vi "Read Test.vi"() -> ()   [LabVIEW 2020]
uses:
  <vilib>/Waveform/WDTOps.llb/WDT Get Waveform Time Array DBL.vi
panel:
  out "x-y 2":dbl
  out "x-y":dbl
  out "XY Graph":cluster{"X array":timestamp[], "Y":dbl[]}(graph)
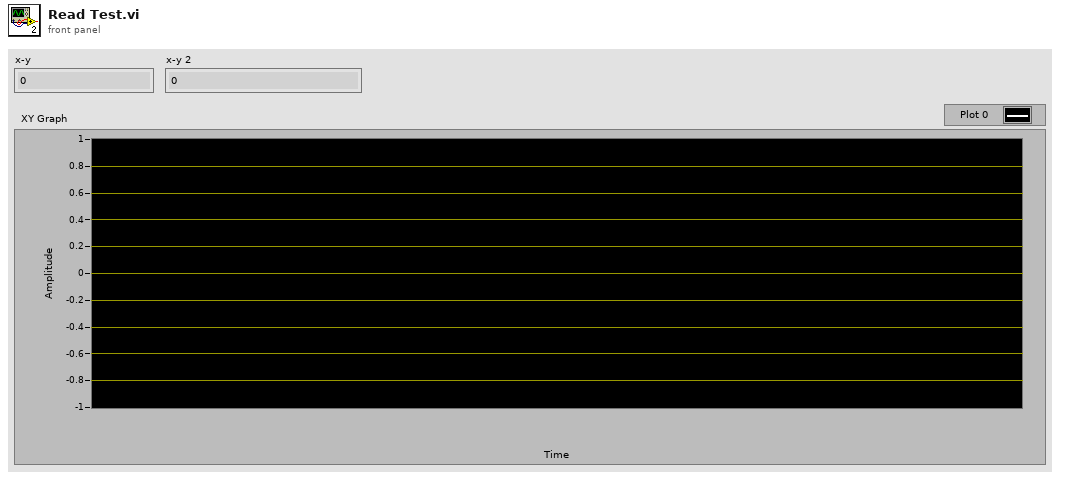
[diagram p1: front panel]
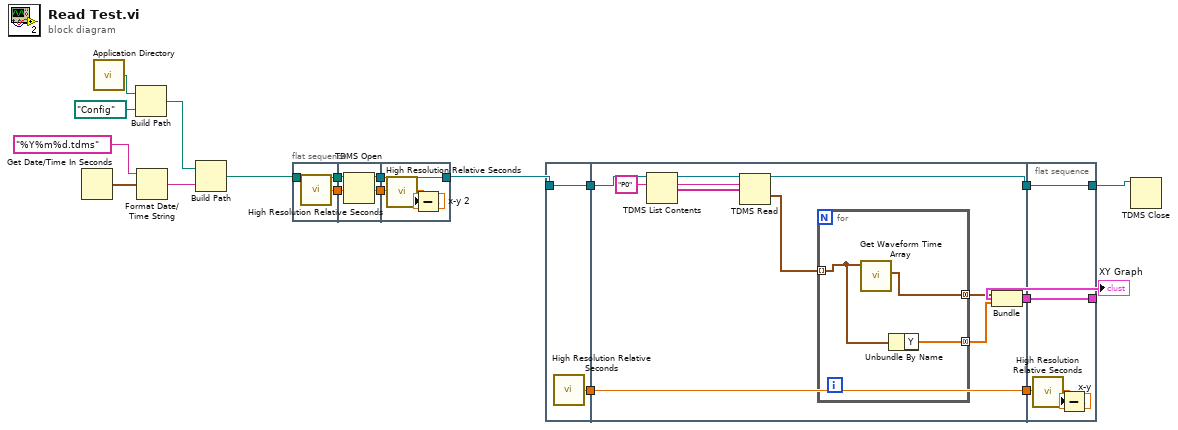
[diagram p0: block diagram]
diagram:
  n1 = Get Date/Time In Seconds() -> (seconds since 1Jan1904=w17:timestamp)
  n2 = call <vilib>:"Application Directory.vi"() -> ("Application Directory"=w19:path)
  n3 = Build Path(base path=w19, name or relative path=path "Config") -> (appended path=w16:path)
  n4 = Format Date/Time String(time format string (%c)="%Y%m%d.tdms", seconds (now)=w17) -> (date/time string=w14:string)  [unwired: 1 in]
  n5 = Build Path(base path=w16, name or relative path=w14) -> (appended path=w13:path)
  n6 = flat-sequence {
    tunnel: w13 -> [w21]
    tunnel: [w21] -> w3
    tunnel: [w20] -> w1
    tunnel: [w23] -> w4
    tunnel: w3 -> [w24]
    tunnel: [w22] -> w2
    tunnel: w1 -> [w22]
    tunnel: [w28] -> w7
    tunnel: w4 -> [w28]
    tunnel: w2 -> [w26]
    frame #0 {
      n7 = call <vilib>:"High Resolution Relative Seconds.vi"() -> ("relative seconds"=w20:dbl)
    }
    frame #1 {
      n8 = TDMS Open(11:w24) -> (3:w23:refnum<k34>)  [unwired: 6 in, 1 out]
    }
    frame #2 {
      n9 = call <vilib>:"High Resolution Relative Seconds.vi"() -> ("relative seconds"=w27:dbl)
      n10 = Subtract(x=w27, y=w26) -> (x-y=→"x-y 2":dbl)
    }
  }
  n11 = flat-sequence {
    tunnel: w7 -> [w30]
    tunnel: [w30] -> w12
    tunnel: [w29] -> w11
    tunnel: [w36] -> w10
    tunnel: [w32] -> w9
    tunnel: w12 -> [w41]
    tunnel: [w31] -> w8
    tunnel: w11 -> [w31]
    tunnel: [w48] -> w6
    tunnel: [w49] -> w5
    tunnel: w10 -> [w49]
    tunnel: w9 -> [w48]
    tunnel: w8 -> [w46]
    frame #0 {
      n12 = call <vilib>:"High Resolution Relative Seconds.vi"() -> ("relative seconds"=w29:dbl)
    }
    frame #1 {
      n13 = TDMS List Contents(6:"P0" ("group name"), 7:w41) -> (1:w37:string[], 2:w38:string, 3:w39:refnum<k34>)  [unwired: 1 in, 1 out]
      n14 = TDMS Read(0:w39, 5:w38, 7:w37) -> (4:w36:refnum<k34>, 10:w35:waveform(dbl)[])  [unwired: 5 in, 4 out]
      n15 = for {
        tunnel: w35 -> [w43] mode=indexing
        tunnel: [w44] -> w34 mode=concatenating
        tunnel: [w42] -> w33 mode=concatenating
        n16 = call-poly <vilib>:"Get Waveform Time Array.vi"("waveform in"=w43) -> ("X array"=w44:timestamp[])  [unwired: 9 in, 1 out]
        n17 = Unbundle By Name(w43) -> ("Y"=w42:dbl[])
      }
      n18 = Bundle("X array"=w34, "Y"=w33) -> (w32:cluster{"X array":timestamp[], "Y":dbl[]})  [unwired: 1 in]
    }
    frame #2 {
      n19 = call <vilib>:"High Resolution Relative Seconds.vi"() -> ("relative seconds"=w47:dbl)
      n20 = Subtract(x=w47, y=w46) -> (x-y=→"x-y":dbl)
    }
  }
  n21 = TDMS Close(11:w5) -> ()  [unwired: 1 in, 2 out]
  "XY Graph" <- w6
